vi "CAENSetPointRamp.vi"(8 "error in (no error)":errorcluster, 9 "Field/Current Ratio":dbl, 10 "Setpoint [T]":dbl, 11 "Network Session":refnum<k5>) -> (0 "error out":errorcluster, 2 "PS Response":string, 3 "Network Session Out":refnum<k5>)   [LabVIEW 2025]
doc: "Author: Scott Hannahs <sth@magnet.fsu.edu>\n\nThis software is licensed for use under the “MIT License\"\nCopyright (c) 2025 Scott Hannahs, sth@sth@magnet.sthnet.net\n\nPermission is hereby granted, free of charge, to any person obtaining a copy of this software and associated documentation files (the \"Software\"), to deal in the Software without restriction, including without limitation the rights to use, copy, modify, merge, publish, distribute, sublicense, and/or sell copies of the Software, and to permit persons to whom the Software is furnished to do so, subject to the following conditions: The above copyright notice and this permission notice shall be included in all copies or substantial portions of the Software.\n\nTHE SOFTWARE IS PROVIDED \"AS IS\", WITHOUT WARRANTY OF ANY KIND, EXPRESS OR IMPLIED, INCLUDING BUT NOT LIMITED TO THE WARRANTIES OF MERCHANTABILITY, FITNESS FOR A PARTICULAR PURPOSE AND NONINFRINGEMENT. IN NO EVENT SHALL THE AUTHORS OR COPYRIGHT HOLDERS BE LIABLE FOR ANY CLAIM, DAMAGES OR OTHER LIABILITY, WHETHER IN AN ACTION OF CONTRACT, TORT OR OTHERWISE, ARISING FROM, OUT OF OR IN CONNECTION WITH THE SOFTWARE OR THE USE OR OTHER DEALINGS IN THE SOFTWARE."
panel:
  out "Setpoint [A]":dbl
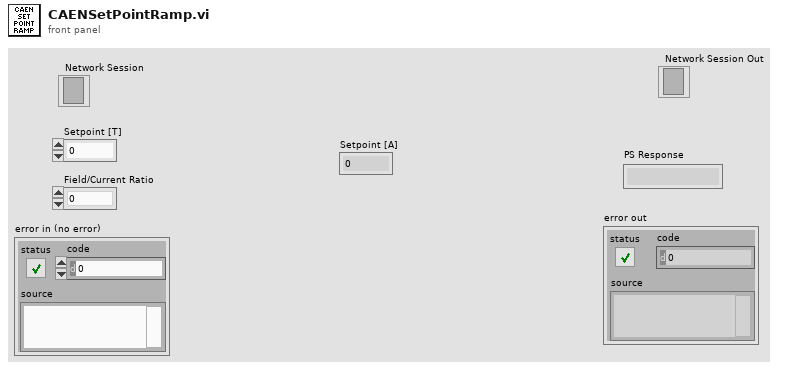
[diagram p1: front panel]
types:
  T1 = enum16{"Standard", "Buffered", "CRLF", "Immediate"}
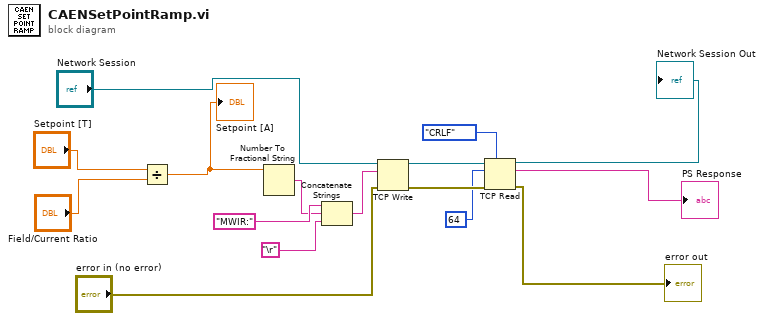
[diagram p0: block diagram]
diagram:
  n1 = Divide(x="Setpoint [T]", y="Field/Current Ratio") -> (x/y=w14:dbl)
  "Setpoint [A]" <- w14
  n2 = Number To Fractional String(number=w14) -> (F-format string=w12:string)  [unwired: 3 in]
  n3 = Concatenate Strings("MWIR:", w12, "\r") -> (w10:string)
  n4 = TCP Write(connection ID="Network Session", data in=w10, error in (no error)="error in (no error)") -> (connection ID out=w5:refnum<k5>, error out=w7:errorcluster)  [unwired: 1 in, 1 out]
  n5 = TCP Read(connection ID=w5, bytes to read=64, error in (no error)=w7, 7:T1."CRLF" ("mode (standard)")) -> (connection ID out=→"Network Session Out":refnum<k5>, data out=→"PS Response":string, error out=→"error out":errorcluster)  [unwired: 1 in]
